vi "Measure_Resistances.vi"(10 "Manual Pressure Set":dbl[](array[numeric])=[400.0, 400.0]) -> (2 "GssDagger":dbl[][](array[numeric]), 3 "R":dbl[](array[numeric]))   [LabVIEW 2016]
uses:
  <userlib>/Fluigent/Fluigent MFCS/FluigentMFCS_Full.llb/MFCS_EZ Detect.vi
  <userlib>/Fluigent/Fluigent MFCS/FluigentMFCS_Full.llb/MFCS_EZ Initialization.vi
  <userlib>/Fluigent/Fluigent MFCS/FluigentMFCS_Full.llb/MFCS_EZ Write Channel Pressure.vi
  <vilib>/imath/engines/lvmath2/RunTimeEngine/IndexReplace/NIMS V(S)=S.vi
  <instcachedir>/0/NIMS V(S)=S_5B9D821375184D3582A2146CD1A04ED7.lvgen/NIMS V(S)=S_5B9D821375184D3582A2146CD1A04ED7_000.vi
  <vilib>/imathl/engines/lvmath/Functions/Error Handling/Create Error.vi
  <vilib>/imath/engines/lvmath2/RunTimeEngine/BuiltInFunctions/length/NIMS_length(GV).vi
  <instcachedir>/0/NIMS_length(GV)_08A3D13377FD4E4B96F5795FBF3698FA.lvgen/NIMS_length(GV)_08A3D13377FD4E4B96F5795FBF3698FA_000.vi
  <vilib>/imath/engines/lvmath2/RunTimeEngine/BuiltInFunctions/reshapemx/NIMS_[GV]_reshapemx.vi
  <instcachedir>/0/NIMS_[GV]_reshapemx_C4E9DBEAD43B49A38F656BB9666BF409.lvgen/NIMS_[GV]_reshapemx_C4E9DBEAD43B49A38F656BB9666BF409_000.vi
  <vilib>/imath/engines/lvmath2/RunTimeEngine/BuiltInFunctions/sum/NIMS_sum(GV).vi
  <instcachedir>/0/NIMS_sum(GV)_67F5EC36BC034E54A6BEC5B0673C00E5.lvgen/NIMS_sum(GV)_67F5EC36BC034E54A6BEC5B0673C00E5_000.vi
  <vilib>/imath/engines/lvmath2/RunTimeEngine/IndexReplace/NIMS M(S,S)=S.vi
  <instcachedir>/0/NIMS M(S,S)=S_EAFF56CDE3BD41B8A97627D4C4AABF63.lvgen/NIMS M(S,S)=S_EAFF56CDE3BD41B8A97627D4C4AABF63_002.vi
  <vilib>/imath/engines/lvmath2/RunTimeEngine/BuiltInFunctions/diag/NIMS_diag.vi
  <instcachedir>/0/NIMS_diag_18AF9B7E8A464F25878B31F262CB73F2.lvgen/NIMS_diag_18AF9B7E8A464F25878B31F262CB73F2_003.vi
  <vilib>/imath/engines/lvmath2/RunTimeEngine/ArithmeticOperatorToken/NIMS_ArithmeticOperator_multmx.vi
  <instcachedir>/0/NIMS_ArithmeticOperator_multmx_B37D95091A3A4016AF0A4F500B490D51.lvgen/NIMS_ArithmeticOperator_multmx_B37D95091A3A4016AF0A4F500B490D51_004.vi
  <vilib>/imath/engines/lvmath2/RunTimeEngine/ArithmeticOperatorToken/NIMS_ArithmeticOperator_plus.vi
  <instcachedir>/0/NIMS_ArithmeticOperator_plus_C66E168CFD7E4B8EADE9B07A37DF7C62.lvgen/NIMS_ArithmeticOperator_plus_C66E168CFD7E4B8EADE9B07A37DF7C62_011.vi
  <vilib>/imath/engines/lvmath2/RunTimeEngine/ErrorHandling/NIMS_Create Error From Enums.vi
  <vilib>/imath/engines/lvmath2/RunTimeEngine/IndexRead/NIMS M(R2,$).vi
  <instcachedir>/0/NIMS M(R2,$)_AD8DC2FC79024024B2717E13B4A0EB4B.lvgen/NIMS M(R2,$)_AD8DC2FC79024024B2717E13B4A0EB4B_000.vi
  <vilib>/imath/engines/lvmath2/RunTimeEngine/ArithmeticOperatorToken/NIMS_ArithmeticOperator_multmx-internal.vi
  <instcachedir>/0/NIMS_ArithmeticOperator_multmx-internal_1F77441B23F34E498AE8F32A2F857701.lvgen/NIMS_ArithmeticOperator_multmx-internal_1F77441B23F34E498AE8F32A2F857701_004.vi
  <vilib>/imath/engines/lvmath2/RunTimeEngine/ArithmeticOperatorToken/NIMS_ArithmeticOperator_rightdivmx-internal.vi
  <instcachedir>/0/NIMS_ArithmeticOperator_rightdivmx-internal_405A11486C6C47468A9656351A7528C1.lvgen/NIMS_ArithmeticOperator_rightdivmx-internal_405A11486C6C47468A9656351A7528C1_000.vi
  <vilib>/imath/engines/lvmath2/RunTimeEngine/NodeEndStatement/NIMS_NodeEndStatement_Output.vi
  <instcachedir>/0/NIMS_NodeEndStatement_Output_53EC0D466D134D7ABD903AC30B43404B.lvgen/NIMS_NodeEndStatement_Output_53EC0D466D134D7ABD903AC30B43404B_002.vi
  <instcachedir>/0/NIMS_NodeEndStatement_Output_53EC0D466D134D7ABD903AC30B43404B.lvgen/NIMS_NodeEndStatement_Output_53EC0D466D134D7ABD903AC30B43404B_005.vi
  <vilib>/imath/engines/lvmath2/RunTimeEngine/ErrorHandling/NIMS_Finalize Error.vi
  Gss.vi
panel:
  in  "Pressure Channels":i16[](array[numeric])=[2, 3]
  in  "Boards":enum16{"A", "B", "C"}[](array[ring])=[enum."A", enum."A"]
  in  "Valves":enum16{"1", "2", "3", "4", "5", "6", "7", "8"}[](array[ring])=[enum."5", enum."1"]
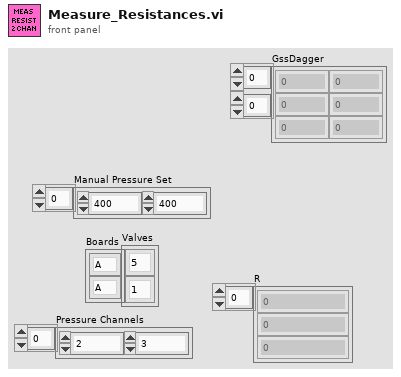
[diagram p1: front panel]
types:
  T1 = typedef "_EZmfcsSN.ctl" = u16
  T2 = typedef "_EZmfcsRefNum.ctl" = refnum<k1>
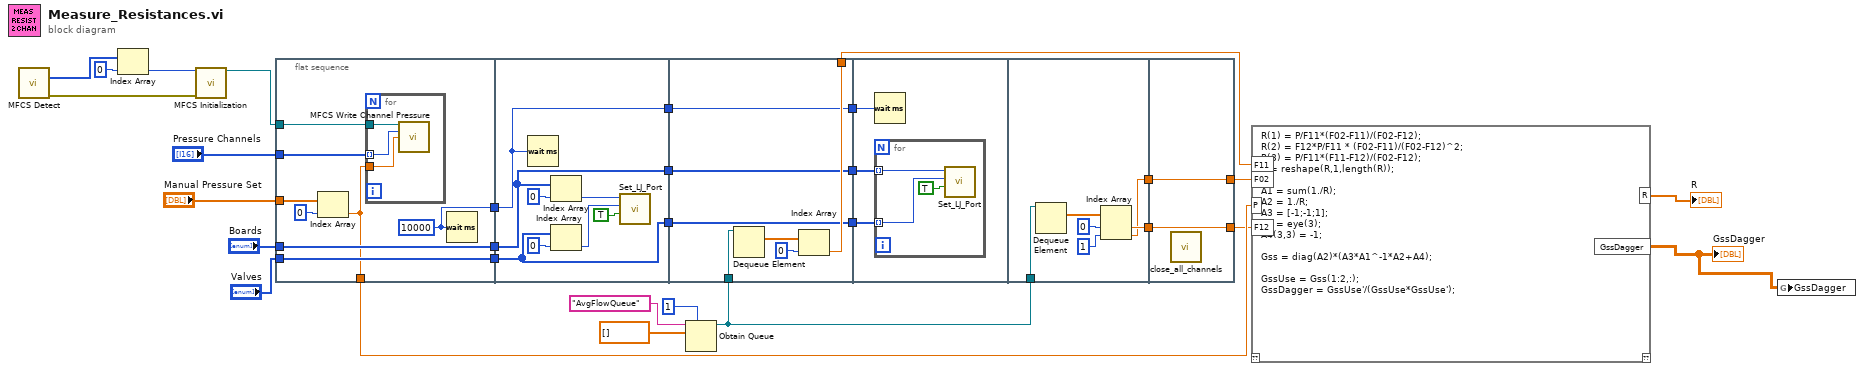
[diagram p0: block diagram]
diagram:
  n1 = call-poly <userlib>:"MFCS Detect.vi"() -> ("[SN MFCS_EZ]"=w27:T1[], "error out"=w25:errorcluster)  [unwired: 14 in]
  n2 = Index Array(array=w27, index=0) -> (element=w26:T1)
  n3 = call-poly <userlib>:"MFCS Initialization.vi"("SN MFCS_EZ"=w26, "error in (no error)"=w25) -> ("MFCS_EZ"=w17:T2)  [unwired: 11 in, 2 out]
  n4 = flat-sequence {
    tunnel: "Boards" -> [w37]
    tunnel: "Valves" -> [w38]
    tunnel: [w38] -> w21
    tunnel: [w37] -> w20
    tunnel: "Manual Pressure Set" -> [w36]
    tunnel: "Pressure Channels" -> [w35]
    tunnel: w17 -> [w34]
    tunnel: [w33] -> w16
    tunnel: [w31] -> w14
    tunnel: w21 -> [w43]
    tunnel: w20 -> [w44]
    tunnel: w16 -> [w42]
    tunnel: [w44] -> w12
    tunnel: [w43] -> w10
    tunnel: [w42] -> w9
    tunnel: w7 -> [w56]
    tunnel: [w53] -> w15
    tunnel: [w52] -> w13
    tunnel: w12 -> [w52]
    tunnel: [w51] -> w11
    tunnel: w10 -> [w51]
    tunnel: w9 -> [w50]
    tunnel: [w50] -> w8
    tunnel: w13 -> [w59]
    tunnel: w11 -> [w58]
    tunnel: w8 -> [w57]
    tunnel: w7 -> [w68]
    tunnel: [w64] -> w4
    tunnel: [w63] -> w3
    tunnel: [w69] -> w5
    tunnel: [w70] -> w6
    tunnel: w4 -> [w70]
    tunnel: w3 -> [w69]
    frame #0 {
      w33 = u32 10000 ("milliseconds to wait")
      n5 = Index Array(array=w36, index=0) -> (element=w31:dbl)
      n6 = for {
        tunnel: w31 -> [w41]
        tunnel: w35 -> [w40] mode=indexing
        tunnel: w34 -> [w39]
        n7 = call-poly <userlib>:"MFCS Write Channel Pressure.vi"("MFCS_EZ"=w39, "Channel Number (default=1)"=w40, "Pressure (mBar)"=w41) -> ()  [unwired: 11 in, 2 out]
      }
      n8 = Wait (ms)(milliseconds to wait=w33) -> ()  [unwired: 1 out]
    }
    frame #1 {
      n9 = Wait (ms)(milliseconds to wait=w42) -> ()  [unwired: 1 out]
      n10 = Index Array(array=w44, index=0) -> (element=w48:enum16{"A", "B", "C"})
      n11 = Index Array(array=w43, index=0) -> (element=w46:enum16{"1", "2", "3", "4", "5", "6", "7", "8"})
      n12 = call "Set_LJ_Port.vi"("State"=TRUE, "Channel"=w46, "Flowboard"=w48) -> ()  [unwired: 8 in, 1 out]
    }
    frame #2 {
      n13 = Dequeue Element(queue=w56) -> (element=w55:dbl[])  [unwired: 2 in, 3 out]
      n14 = Index Array(array=w55, index=0) -> (element=w53:dbl)
    }
    frame #3 {
      n15 = Wait (ms)(milliseconds to wait=w57) -> ()  [unwired: 1 out]
      n16 = for {
        tunnel: w59 -> [w61] mode=indexing
        tunnel: w58 -> [w60] mode=indexing
        n17 = call "Set_LJ_Port.vi"("State"=TRUE, "Channel"=w60, "Flowboard"=w61) -> ()  [unwired: 8 in, 1 out]
      }
    }
    frame #4 {
      n18 = Dequeue Element(queue=w68) -> (element=w67:dbl[])  [unwired: 2 in, 3 out]
      n19 = Index Array(array=w67, index #1=0 ("index"), index #2=1 ("index")) -> (element #1=w64:dbl, element #2=w63:dbl)
    }
    frame #5 {
      n20 = call "close_all_channels.vi"() -> ()  [unwired: 12 in]
    }
  }
  n21 = Obtain Queue(max queue size (-1, unlimited)=1, name (unnamed)="AvgFlowQueue", element data type=dbl[] [] ("appended array")) -> (queue out=w7:refnum<queue>)  [unwired: 2 in, 2 out]
  n22 = mathscript code="R(1) = P/F11*(F02-F11)/(F02-F12);\nR(2) = F12*P/F11 * (F02-F11)/(F02-F12)^2;\nR(3) = P/F11*(F11-F12)/(F02-F12);\nR = reshape(R,1,length(R));\n\nA1 = sum(1./R);\nA2 = 1./R;\nA3 = [-1;-1;1];\nA4 = eye(3);\nA4(3,3) = -1;\n\nGss = diag(A2)*(A3*A1^-1*A2+A4);\n\nGssUse = Gss(1:2,:);\nGssDagger = GssUse'/(GssUse*GssUse');"("P"=w14, "F11"=w15, "F02"=w5, "F12"=w6) -> ("R"=→"R":dbl[], "GssDagger"=w1:dbl[][])  [unwired: 1 in, 1 out]
  "GssDagger" <- w1
  n23 = global write "Gss.vi" "GssDagger"(w1) -> ()
